vi "get cursor win.vi"(4 "right":dbl, 6 "left":dbl, 10 "freq":dbl[](array[numeric])=[0.0, 2.033333331346512, 4.066666662693024, 6.0999999940395355, 8.133333332836628, 14.83333332836628, 21.516666665673256, 28.216666661202908, 29.25, 30.283333331346512, 32.04999999701977, 33.08333332836628, 34.099999994039536, 35.13333333283663, 36.16666666418314, 37.19999999552965, 38.21666666120291, 39.25, 40.28333333134651, 41.316666662693024, 42.349999994039536, 43.36666665971279, 44.399999998509884, 45.433333329856396, 46.46666666120291, 47.48333332687616, 48.516666665673256, 49.54999999701977, 50.58333332836628, 51.599999994039536, 52.63333333283663, 53.66666666418314, 54.69999999552965, 55.71666666120291, 56.75, 57.78333333134651, 58.816666662693024, 59.849999994039536, 60.86666665971279, 61.899999998509884, 62.933333329856396, 63.96666666120291, 64.98333332687616, 66.01666666567326, 67.04999999701977, 68.08333332836628, 69.09999999403954, 70.13333333283663, 71.16666666418314, 72.19999999552965, 73.21666666120291, 74.25, 75.28333333134651, 76.31666666269302, 77.33333332836628, 78.36666665971279, 79.39999999850988, 80.4333333298564, 81.46666666120291, 82.48333332687616, 83.51666666567326, 84.54999999701977, 85.58333332836628, 86.61666665971279, 87.63333333283663, 88.66666666418314, 89.69999999552965, 90.73333332687616, 91.75, 92.78333333134651, 93.81666666269302, 94.84999999403954, 95.88333333283663, 96.89999999850988, 97.9333333298564, 98.96666666120291, 100.0, 101.03333333134651, 102.04999999701977, 103.08333332836628, 104.11666665971279, 105.14999999850988, 106.16666666418314, 107.19999999552965, 108.23333332687616, 109.26666666567326, 110.29999999701977, 111.31666666269302, 112.34999999403954, 113.38333333283663, 114.41666666418314, 115.44999999552965, 116.46666666120291, 117.5, 118.53333333134651, 119.56666666269302, 120.59999999403954, 121.61666665971279, 122.64999999850988, 123.6833333298564, 124.71666666120291, 125.73333332687616, 126.76666666567326, 127.79999999701977, 128.83333332836628, 129.84999999403954, 130.88333333283663, 131.91666666418314, 132.94999999552965, 133.98333332687616, 135.0, 136.0333333313465, 137.06666666269302, 138.09999999403954, 139.13333333283663, 140.16666666418314, 141.19999999552965, 142.23333332687616, 143.25, 144.2833333313465, 145.31666666269302, 146.34999999403954, 147.38333333283663, 148.41666666418314, 149.4333333298564, 150.4666666612029, 151.5, 152.5333333313465, 153.56666666269302, 154.58333332836628, 155.6166666597128, 156.64999999850988, 157.6833333298564, 158.69999999552965, 159.73333332687616, 160.76666666567326, 161.79999999701977, 162.83333332836628, 163.84999999403954, 164.88333333283663, 165.91666666418314, 166.94999999552965, 167.98333332687616, 169.0, 170.0333333313465, 171.06666666269302, 172.09999999403954, 173.13333333283663, 174.14999999850988, 175.1833333298564, 176.2166666612029, 177.25, 178.26666666567326, 179.29999999701977, 180.33333332836628, 181.3666666597128, 182.39999999850988, 183.41666666418314, 184.44999999552965, 185.48333332687616, 186.51666666567326, 187.54999999701977, 188.56666666269302, 189.59999999403954, 190.63333333283663, 191.66666666418314, 192.69999999552965, 193.7166666612029, 194.75, 195.7833333313465, 196.81666666269302, 197.84999999403954, 198.8666666597128, 199.89999999850988, 200.9333333298564, 201.9666666612029, 202.98333332687616, 204.01666666567326, 205.04999999701977, 206.08333332836628, 207.1166666597128, 208.13333333283663, 209.16666666418314, 210.19999999552965, 211.23333332687616, 212.25, 213.2833333313465, 214.31666666269302, 215.34999999403954, 216.38333333283663, 217.39999999850988, 218.4333333298564, 219.4666666612029, 220.5, 221.5333333313465, 222.54999999701977, 223.58333332836628, 224.6166666597128, 225.64999999850988, 226.6833333298564, 227.69999999552965, 228.73333332687616, 229.76666666567326, 230.79999999701977, 231.81666666269302, 232.84999999403954, 233.88333333283663, 234.91666666418314, 235.94999999552965, 236.9666666612029, 238.0, 239.0333333313465, 240.06666666269302, 241.08333332836628, 242.1166666597128, 243.14999999850988, 244.1833333298564, 245.2166666612029, 246.23333332687616, 247.26666666567326, 248.29999999701977, 249.33333332836628, 250.34999999403954, 251.38333333283663, 252.41666666418314, 253.44999999552965, 254.48333332687616, 255.5, 256.5333333313465, 257.566666662693, 258.59999999403954, 259.6166666597128, 260.6499999985099, 261.6833333298564, 262.7166666612029, 263.75, 264.76666666567326, 265.79999999701977, 266.8333333283663, 267.8666666597128, 268.8999999985099, 269.91666666418314, 270.94999999552965, 271.98333332687616, 273.01666666567326, 274.04999999701977, 275.066666662693, 276.09999999403954, 277.1333333328366, 278.16666666418314, 279.19999999552965, 280.2166666612029, 281.25, 282.2833333313465, 283.316666662693, 284.34999999403954, 285.3666666597128, 286.3999999985099, 287.4333333298564, 288.4666666612029, 289.48333332687616, 290.51666666567326, 291.54999999701977, 292.5833333283663, 293.6166666597128, 294.6333333328366, 295.66666666418314, 296.69999999552965, 297.73333332687616, 298.75, 299.7833333313465, 300.816666662693, 301.84999999403954, 302.8833333328366, 303.8999999985099, 304.9333333298564, 305.9666666612029, 307.0, 308.0333333313465, 309.04999999701977, 310.0833333283663, 311.1166666597128, 312.1499999985099, 313.16666666418314, 314.19999999552965, 315.23333332687616, 316.26666666567326, 317.29999999701977, 318.316666662693, 319.34999999403954, 320.3833333328366, 321.41666666418314, 322.4333333298564, 323.4666666612029, 324.5, 325.5333333313465, 326.566666662693, 327.5833333283663, 328.6166666597128, 329.6499999985099, 330.6833333298564, 331.69999999552965, 332.73333332687616, 333.76666666567326, 334.79999999701977, 335.8333333283663, 336.84999999403954, 337.8833333328366, 338.91666666418314, 339.94999999552965, 340.98333332687616, 342.0, 343.0333333313465, 344.066666662693, 345.09999999403954, 346.1166666597128], 11 "time points":dbl[](array[numeric])=[0.0, 2.033333331346512, 4.066666662693024, 6.0999999940395355, 8.133333332836628, 14.83333332836628, 21.516666665673256, 28.216666661202908, 29.25, 30.283333331346512, 32.04999999701977, 33.08333332836628, 34.099999994039536, 35.13333333283663, 36.16666666418314, 37.19999999552965, 38.21666666120291, 39.25, 40.28333333134651, 41.316666662693024, 42.349999994039536, 43.36666665971279, 44.399999998509884, 45.433333329856396, 46.46666666120291, 47.48333332687616, 48.516666665673256, 49.54999999701977, 50.58333332836628, 51.599999994039536, 52.63333333283663, 53.66666666418314, 54.69999999552965, 55.71666666120291, 56.75, 57.78333333134651, 58.816666662693024, 59.849999994039536, 60.86666665971279, 61.899999998509884, 62.933333329856396, 63.96666666120291, 64.98333332687616, 66.01666666567326, 67.04999999701977, 68.08333332836628, 69.09999999403954, 70.13333333283663, 71.16666666418314, 72.19999999552965, 73.21666666120291, 74.25, 75.28333333134651, 76.31666666269302, 77.33333332836628, 78.36666665971279, 79.39999999850988, 80.4333333298564, 81.46666666120291, 82.48333332687616, 83.51666666567326, 84.54999999701977, 85.58333332836628, 86.61666665971279, 87.63333333283663, 88.66666666418314, 89.69999999552965, 90.73333332687616, 91.75, 92.78333333134651, 93.81666666269302, 94.84999999403954, 95.88333333283663, 96.89999999850988, 97.9333333298564, 98.96666666120291, 100.0, 101.03333333134651, 102.04999999701977, 103.08333332836628, 104.11666665971279, 105.14999999850988, 106.16666666418314, 107.19999999552965, 108.23333332687616, 109.26666666567326, 110.29999999701977, 111.31666666269302, 112.34999999403954, 113.38333333283663, 114.41666666418314, 115.44999999552965, 116.46666666120291, 117.5, 118.53333333134651, 119.56666666269302, 120.59999999403954, 121.61666665971279, 122.64999999850988, 123.6833333298564, 124.71666666120291, 125.73333332687616, 126.76666666567326, 127.79999999701977, 128.83333332836628, 129.84999999403954, 130.88333333283663, 131.91666666418314, 132.94999999552965, 133.98333332687616, 135.0, 136.0333333313465, 137.06666666269302, 138.09999999403954, 139.13333333283663, 140.16666666418314, 141.19999999552965, 142.23333332687616, 143.25, 144.2833333313465, 145.31666666269302, 146.34999999403954, 147.38333333283663, 148.41666666418314, 149.4333333298564, 150.4666666612029, 151.5, 152.5333333313465, 153.56666666269302, 154.58333332836628, 155.6166666597128, 156.64999999850988, 157.6833333298564, 158.69999999552965, 159.73333332687616, 160.76666666567326, 161.79999999701977, 162.83333332836628, 163.84999999403954, 164.88333333283663, 165.91666666418314, 166.94999999552965, 167.98333332687616, 169.0, 170.0333333313465, 171.06666666269302, 172.09999999403954, 173.13333333283663, 174.14999999850988, 175.1833333298564, 176.2166666612029, 177.25, 178.26666666567326, 179.29999999701977, 180.33333332836628, 181.3666666597128, 182.39999999850988, 183.41666666418314, 184.44999999552965, 185.48333332687616, 186.51666666567326, 187.54999999701977, 188.56666666269302, 189.59999999403954, 190.63333333283663, 191.66666666418314, 192.69999999552965, 193.7166666612029, 194.75, 195.7833333313465, 196.81666666269302, 197.84999999403954, 198.8666666597128, 199.89999999850988, 200.9333333298564, 201.9666666612029, 202.98333332687616, 204.01666666567326, 205.04999999701977, 206.08333332836628, 207.1166666597128, 208.13333333283663, 209.16666666418314, 210.19999999552965, 211.23333332687616, 212.25, 213.2833333313465, 214.31666666269302, 215.34999999403954, 216.38333333283663, 217.39999999850988, 218.4333333298564, 219.4666666612029, 220.5, 221.5333333313465, 222.54999999701977, 223.58333332836628, 224.6166666597128, 225.64999999850988, 226.6833333298564, 227.69999999552965, 228.73333332687616, 229.76666666567326, 230.79999999701977, 231.81666666269302, 232.84999999403954, 233.88333333283663, 234.91666666418314, 235.94999999552965, 236.9666666612029, 238.0, 239.0333333313465, 240.06666666269302, 241.08333332836628, 242.1166666597128, 243.14999999850988, 244.1833333298564, 245.2166666612029, 246.23333332687616, 247.26666666567326, 248.29999999701977, 249.33333332836628, 250.34999999403954, 251.38333333283663, 252.41666666418314, 253.44999999552965, 254.48333332687616, 255.5, 256.5333333313465, 257.566666662693, 258.59999999403954, 259.6166666597128, 260.6499999985099, 261.6833333298564, 262.7166666612029, 263.75, 264.76666666567326, 265.79999999701977, 266.8333333283663, 267.8666666597128, 268.8999999985099, 269.91666666418314, 270.94999999552965, 271.98333332687616, 273.01666666567326, 274.04999999701977, 275.066666662693, 276.09999999403954, 277.1333333328366, 278.16666666418314, 279.19999999552965, 280.2166666612029, 281.25, 282.2833333313465, 283.316666662693, 284.34999999403954, 285.3666666597128, 286.3999999985099, 287.4333333298564, 288.4666666612029, 289.48333332687616, 290.51666666567326, 291.54999999701977, 292.5833333283663, 293.6166666597128, 294.6333333328366, 295.66666666418314, 296.69999999552965, 297.73333332687616, 298.75, 299.7833333313465, 300.816666662693, 301.84999999403954, 302.8833333328366, 303.8999999985099, 304.9333333298564, 305.9666666612029, 307.0, 308.0333333313465, 309.04999999701977, 310.0833333283663, 311.1166666597128, 312.1499999985099, 313.16666666418314, 314.19999999552965, 315.23333332687616, 316.26666666567326, 317.29999999701977, 318.316666662693, 319.34999999403954, 320.3833333328366, 321.41666666418314, 322.4333333298564, 323.4666666612029, 324.5, 325.5333333313465, 326.566666662693, 327.5833333283663, 328.6166666597128, 329.6499999985099, 330.6833333298564, 331.69999999552965, 332.73333332687616, 333.76666666567326, 334.79999999701977, 335.8333333283663, 336.84999999403954, 337.8833333328366, 338.91666666418314, 339.94999999552965, 340.98333332687616, 342.0, 343.0333333313465, 344.066666662693, 345.09999999403954, 346.1166666597128]) -> (2 "freq out":dbl[](array[numeric])=[0.0, 2.033333331346512, 4.066666662693024, 6.0999999940395355, 8.133333332836628, 14.83333332836628, 21.516666665673256, 28.216666661202908, 29.25, 30.283333331346512, 32.04999999701977, 33.08333332836628, 34.099999994039536, 35.13333333283663, 36.16666666418314, 37.19999999552965, 38.21666666120291, 39.25, 40.28333333134651, 41.316666662693024, 42.349999994039536, 43.36666665971279, 44.399999998509884, 45.433333329856396, 46.46666666120291, 47.48333332687616, 48.516666665673256, 49.54999999701977, 50.58333332836628, 51.599999994039536, 52.63333333283663, 53.66666666418314, 54.69999999552965, 55.71666666120291, 56.75, 57.78333333134651, 58.816666662693024, 59.849999994039536, 60.86666665971279, 61.899999998509884, 62.933333329856396, 63.96666666120291, 64.98333332687616, 66.01666666567326, 67.04999999701977, 68.08333332836628, 69.09999999403954, 70.13333333283663, 71.16666666418314, 72.19999999552965, 73.21666666120291, 74.25, 75.28333333134651, 76.31666666269302, 77.33333332836628, 78.36666665971279, 79.39999999850988, 80.4333333298564, 81.46666666120291, 82.48333332687616, 83.51666666567326, 84.54999999701977, 85.58333332836628, 86.61666665971279, 87.63333333283663, 88.66666666418314, 89.69999999552965, 90.73333332687616, 91.75, 92.78333333134651, 93.81666666269302, 94.84999999403954, 95.88333333283663, 96.89999999850988, 97.9333333298564, 98.96666666120291, 100.0, 101.03333333134651, 102.04999999701977, 103.08333332836628, 104.11666665971279, 105.14999999850988, 106.16666666418314, 107.19999999552965, 108.23333332687616, 109.26666666567326, 110.29999999701977, 111.31666666269302, 112.34999999403954, 113.38333333283663, 114.41666666418314, 115.44999999552965, 116.46666666120291, 117.5, 118.53333333134651, 119.56666666269302, 120.59999999403954, 121.61666665971279, 122.64999999850988, 123.6833333298564, 124.71666666120291, 125.73333332687616, 126.76666666567326, 127.79999999701977, 128.83333332836628, 129.84999999403954, 130.88333333283663, 131.91666666418314, 132.94999999552965, 133.98333332687616, 135.0, 136.0333333313465, 137.06666666269302, 138.09999999403954, 139.13333333283663, 140.16666666418314, 141.19999999552965, 142.23333332687616, 143.25, 144.2833333313465, 145.31666666269302, 146.34999999403954, 147.38333333283663, 148.41666666418314, 149.4333333298564, 150.4666666612029, 151.5, 152.5333333313465, 153.56666666269302, 154.58333332836628, 155.6166666597128, 156.64999999850988, 157.6833333298564, 158.69999999552965, 159.73333332687616, 160.76666666567326, 161.79999999701977, 162.83333332836628, 163.84999999403954, 164.88333333283663, 165.91666666418314, 166.94999999552965, 167.98333332687616, 169.0, 170.0333333313465, 171.06666666269302, 172.09999999403954, 173.13333333283663, 174.14999999850988, 175.1833333298564, 176.2166666612029, 177.25, 178.26666666567326, 179.29999999701977, 180.33333332836628, 181.3666666597128, 182.39999999850988, 183.41666666418314, 184.44999999552965, 185.48333332687616, 186.51666666567326, 187.54999999701977, 188.56666666269302, 189.59999999403954, 190.63333333283663, 191.66666666418314, 192.69999999552965, 193.7166666612029, 194.75, 195.7833333313465, 196.81666666269302, 197.84999999403954, 198.8666666597128, 199.89999999850988, 200.9333333298564, 201.9666666612029, 202.98333332687616, 204.01666666567326, 205.04999999701977, 206.08333332836628, 207.1166666597128, 208.13333333283663, 209.16666666418314, 210.19999999552965, 211.23333332687616, 212.25, 213.2833333313465, 214.31666666269302, 215.34999999403954, 216.38333333283663, 217.39999999850988, 218.4333333298564, 219.4666666612029, 220.5, 221.5333333313465, 222.54999999701977, 223.58333332836628, 224.6166666597128, 225.64999999850988, 226.6833333298564, 227.69999999552965, 228.73333332687616, 229.76666666567326, 230.79999999701977, 231.81666666269302, 232.84999999403954, 233.88333333283663, 234.91666666418314, 235.94999999552965, 236.9666666612029, 238.0, 239.0333333313465, 240.06666666269302, 241.08333332836628, 242.1166666597128, 243.14999999850988, 244.1833333298564, 245.2166666612029, 246.23333332687616, 247.26666666567326, 248.29999999701977, 249.33333332836628, 250.34999999403954, 251.38333333283663, 252.41666666418314, 253.44999999552965, 254.48333332687616, 255.5, 256.5333333313465, 257.566666662693, 258.59999999403954, 259.6166666597128, 260.6499999985099, 261.6833333298564, 262.7166666612029, 263.75, 264.76666666567326, 265.79999999701977, 266.8333333283663, 267.8666666597128, 268.8999999985099, 269.91666666418314, 270.94999999552965, 271.98333332687616, 273.01666666567326, 274.04999999701977, 275.066666662693, 276.09999999403954, 277.1333333328366, 278.16666666418314, 279.19999999552965, 280.2166666612029, 281.25, 282.2833333313465, 283.316666662693, 284.34999999403954, 285.3666666597128, 286.3999999985099, 287.4333333298564, 288.4666666612029, 289.48333332687616, 290.51666666567326, 291.54999999701977, 292.5833333283663, 293.6166666597128, 294.6333333328366, 295.66666666418314, 296.69999999552965, 297.73333332687616, 298.75, 299.7833333313465, 300.816666662693, 301.84999999403954, 302.8833333328366, 303.8999999985099, 304.9333333298564, 305.9666666612029, 307.0, 308.0333333313465, 309.04999999701977, 310.0833333283663, 311.1166666597128, 312.1499999985099, 313.16666666418314, 314.19999999552965, 315.23333332687616, 316.26666666567326, 317.29999999701977, 318.316666662693, 319.34999999403954, 320.3833333328366, 321.41666666418314, 322.4333333298564, 323.4666666612029, 324.5, 325.5333333313465, 326.566666662693, 327.5833333283663, 328.6166666597128, 329.6499999985099, 330.6833333298564, 331.69999999552965, 332.73333332687616, 333.76666666567326, 334.79999999701977, 335.8333333283663, 336.84999999403954, 337.8833333328366, 338.91666666418314, 339.94999999552965, 340.98333332687616, 342.0, 343.0333333313465, 344.066666662693, 345.09999999403954, 346.1166666597128])   [LabVIEW 2015]
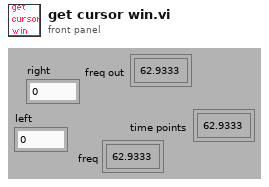
[diagram p1: front panel]
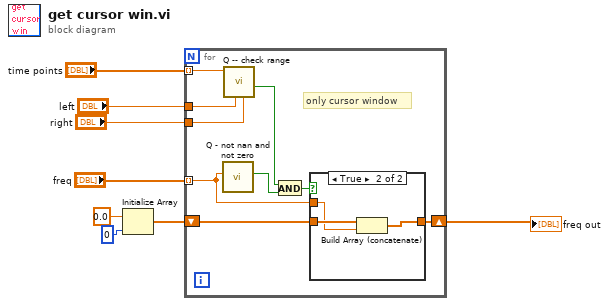
[diagram p0: block diagram]
diagram:
  n1 = Initialize Array(0.0, 0) -> (w2:dbl[])
  n2 = for {
    shift-right: [w16] -> w1
    shift-left: w2 -> [w17]
    tunnel: "freq" -> [w10] mode=indexing
    tunnel: "time points" -> [w14] mode=indexing
    tunnel: "left" -> [w13]
    tunnel: "right" -> [w12]
    # "only cursor window"
    n3 = call "Q - not nan and not zero.vi"("Numeric"=w10) -> ("Boolean"=w11:bool)  [unwired: 10 in]
    n4 = call "Q -- check range.vi"("upper"=w12, "lower"=w13, "number"=w14) -> ("in range?"=w9:bool)  [unwired: 4 in, 4 out]
    n5 = And(x=w9, y=w11) -> (x .and. y?=w15:bool)
    n6 = case shown="True" w15 {
      tunnel: w17 -> [w18 w21]
      tunnel: [w18 w20] -> w16
      tunnel: w10 -> [_ w19]
      frame False {
      }
      frame True {
        n7 = Build Array (concatenate)(w21, w19) -> (w20:dbl[])
      }
    }
  }
  "freq out" <- w1
